vi "XIPIN_Video_PHY_Controller_2_0.vi"   [LabVIEW 2017]
doc: "Video PHY Controller\n------------------------------------\n<b>Need License</b> : No\n<b>Interface</b> : AXI4 AXI4-Stream"
uses:
  <vilib>/rvi/XilinxIP/XIPIN_XNode/niFpgaXIPIN.xnode
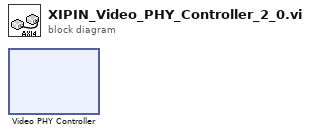
[diagram p0: block diagram]
diagram:
  n1 = xnode ("Video PHY Controller")() -> ()
